vi "BK Precision 911X Series Setup List Program.vi"() -> ()   [LabVIEW 2020]
doc: "This example demonstrates how to setup and save a list program to the internal memory of the instrument."
uses:
  BK Precision 911X Series.lvlib
panel:
  in  "Sequence Repeat Count":i32[](array[numeric])=[1, 1, 1, 1, 1, 1, 1, 1, 1, 1] min=1 max=65535 step=1
  in  "List Power Limit (1200)":dbl=1200.0 min=1.0 max=1200.0 step=1.0
  in  "Linked Sequences (0000000000)":bool[](array[boolean])=[FALSE, FALSE, FALSE, FALSE, FALSE, FALSE, FALSE, FALSE, FALSE, FALSE]
  in  "Repeat Count (1)":i32=1 min=1 max=65535 step=1
  in  "List File Number (1)":dbl=1.0 min=1.0 max=10.0 step=1.0
  in  "VISA resource name":refnum<visa-resource-name>
  # "(c) 2013 B&K Precision Corporation.  ALL RIGHTS RESERVED."
  # "Enter the number of times to repeat each sequence in the Sequence Repeat Count array.  Index 0 is for repeat count for sequence 1, Index 1 for sequence 2,\n... and so on to Index 9 for sequence 10.  If the sequence is not enabled from the Linked Sequences control, the value will still be stored into the instrument's internal memory."
  # "Sequence 1"
  # "Sequence 2"
  # "Sequence 3"
  # "Sequence 4"
  # "Sequence 5"
  # "Sequence 6"
  # "Sequence 7"
  # "Sequence 8"
  # "Sequence 9"
  # "Sequence 10"
  # "Sequence #  1   2    3   4    5   6   7    8   9   0"
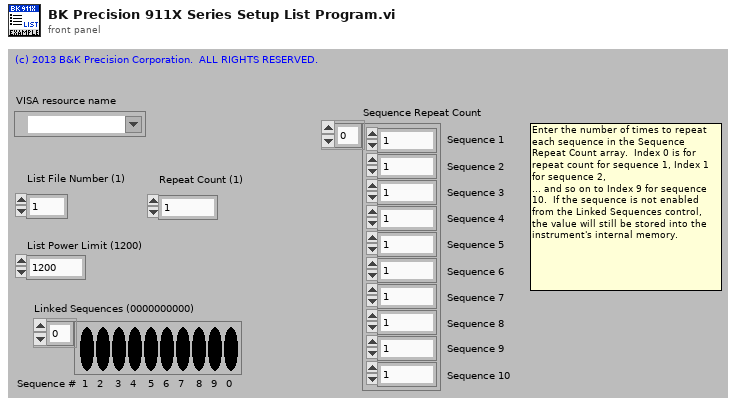
[diagram p1: front panel]
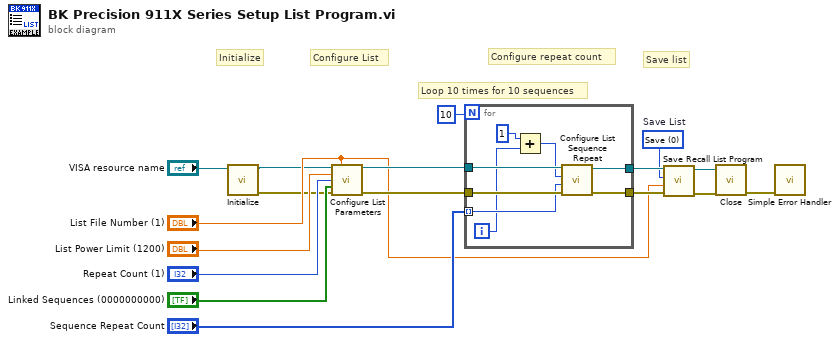
[diagram p0: block diagram]
diagram:
  w4 = u16 0 items=["Save", "Recall"]  # Save List
  # "Loop 10 times for 10 sequences"
  # "Save list"
  # "Configure repeat count"
  # "Configure List"
  # "Initialize"
  n1 = call "Initialize.vi"("VISA resource name"="VISA resource name") -> ("error out"=w1:errorcluster, "VISA resource name out"=w2:refnum<visa-resource-name>)  [unwired: 9 in]
  n2 = call "Configure List Parameters.vi"("VISA resource name"=w2, "List File Number (1)"="List File Number (1)", "List Power Limit (1200)"="List Power Limit (1200)", "Repeat Count (1)"="Repeat Count (1)", "Linked Sequences (0000000000)"="Linked Sequences (0000000000)", "error in (no error)"=w1) -> ("VISA resource name out"=w14:refnum<visa-resource-name>, "error out"=w15:errorcluster)  [unwired: 8 in]
  n3 = for {
    N: 10 -> [_]
    tunnel: w15 -> [w25]
    tunnel: w14 -> [w24]
    tunnel: [w23] -> w13
    tunnel: [w22] -> w12
    tunnel: "Sequence Repeat Count" -> [w21] mode=indexing
    i -> [w19]
    n4 = Add(x=1, y=w19) -> (x+y=w18:i32)
    n5 = call "Configure List Sequence Repeat.vi"("error in (no error)"=w25, "Repeat Count (1)"=w21, "Sequence Number (1)"=w18, "VISA resource name"=w24) -> ("error out"=w22:errorcluster, "VISA resource name out"=w23:refnum<visa-resource-name>)  [unwired: 6 in]
  }
  n6 = call "Save Recall List Program.vi"("error in (no error)"=w12, "List Number (1)"="List File Number (1)", "Save Recall List File (0:Save)"=w4, "VISA resource name"=w13) -> ("error out"=w11:errorcluster, "VISA resource name out"=w10:refnum<visa-resource-name>)  [unwired: 6 in]
  n7 = call "Close.vi"("error in (no error)"=w11, "VISA resource name"=w10) -> ("error out"=w17:errorcluster)  [unwired: 9 in]
  n8 = call <vilib>:"Simple Error Handler.vi"("error in (no error)"=w17) -> ()  [unwired: 4 in, 5 out]
